vi "AlliGator Get Python Function Parameter Values Dialog.vi"(8 "Error In":errorcluster, 10 "Parameters In":string[][](array[string]), 11 "Input Message":string) -> (0 "Error Out":errorcluster, 1 "Cancelled?":bool, 2 "Parameters Out":string[][](array[string]))   [LabVIEW 2021, in "AlliGator Python Plugins.lvlib"]
doc: "Dialog to allow user to enter python function parameters."
uses:
  AlliGator Python Plugins.lvlib
  <vilib>/Utility/error.llb/Error Cluster From Error Code.vi
  <vilib>/ErrorRing/Error Ring.xnode
panel:
  out "Message":string
  in  "Parameters":i32(listbox)
  in  "Cancel":bool
  in  "OK":bool
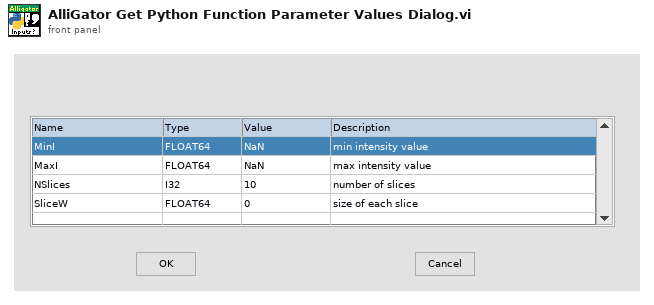
[diagram p1: front panel]
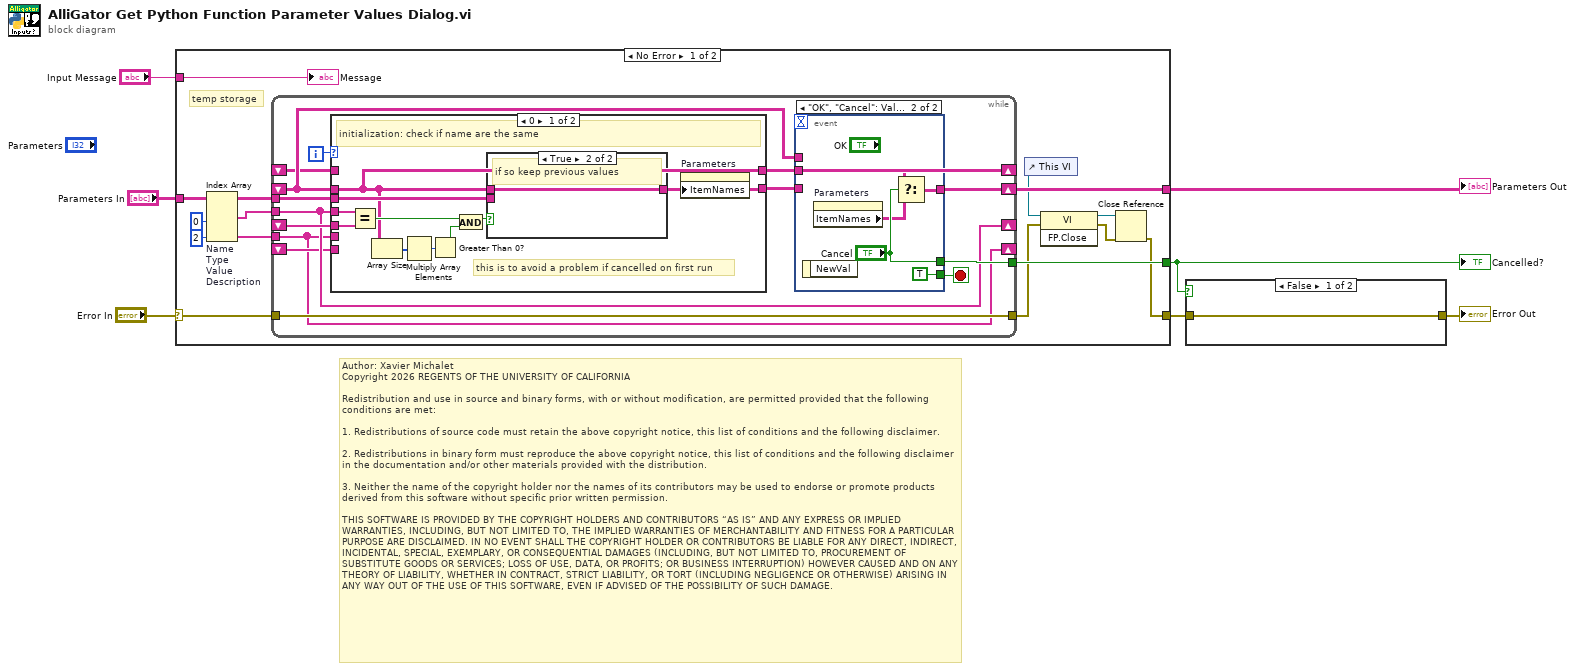
[diagram p0: block diagram]
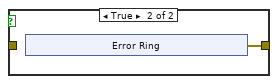
[diagram p2: hidden frame]
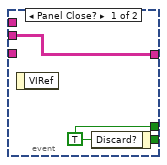
[diagram p5: hidden frame]
diagram:
  # "Author: Xavier Michalet\nCopyright 2026 REGENTS OF THE UNIVERSITY OF CALIFORNIA\n\nRedistribution and use in source and binary forms, with or without modification, are permitted provided that the following conditions are met:\n\n1. Redistributions of source code must retain the above copyright notice, this list of conditions and the following disclaimer.\n\n2. Redistributions in binary form must reproduce the above copyright notice, this list of conditions and the following disclaimer in the documentation and/or other materials provided with the distribution.\n\n3. Neither the name of the copyright holder nor the names of its contributors may be used to endorse or promote products derived from this software without specific prior written permission.\n\nTHIS SOFTWARE IS PROVIDED BY THE COPYRIGHT HOLDERS AND CONTRIBUTORS “AS IS” AND ANY EXPRESS OR IMPLIED WARRANTIES, INCLUDING, BUT NOT LIMITED TO, THE IMPLIED WARRANTIES OF MERCHANTABILITY AND FITNESS FOR A PARTICULAR PURPOSE ARE DISCLAIMED. IN NO EVENT SHALL THE COPYRIGHT HOLDER OR CONTRIBUTORS BE LIABLE FOR ANY DIRECT, INDIRECT, INCIDENTAL, SPECIAL, EXEMPLARY, OR CONSEQUENTIAL DAMAGES (INCLUDING, BUT NOT LIMITED TO, PROCUREMENT OF SUBSTITUTE GOODS OR SERVICES; LOSS OF USE, DATA, OR PROFITS; OR BUSINESS INTERRUPTION) HOWEVER CAUSED AND ON ANY THEORY OF LIABILITY, WHETHER IN CONTRACT, STRICT LIABILITY, OR TORT (INCLUDING NEGLIGENCE OR OTHERWISE) ARISING IN ANY WAY OUT OF THE USE OF THIS SOFTWARE, EVEN IF ADVISED OF THE POSSIBILITY OF SUCH DAMAGE."
  n1 = case shown="No Error" "Error In" {
    selector: "Error In" -> [w15 w57]
    tunnel: [w21 _] -> w3
    tunnel: [w20 _] -> w4
    tunnel: "Input Message" -> [w19 _]
    tunnel: [w16 w57] -> w2
    tunnel: "Parameters In" -> [w8 _]
    frame No Error {
      # "temp storage"
      n2 = Index Array "Name\nType\nValue\nDescription"(array=w8, index (col) #1=0 ("disabled index (col)"), index (col) #2=2 ("index (col)")) -> (element #1=w10:string[], element #2=w9:string[])  [unwired: 2 in]
      n3 = while {
        tunnel: [w34] -> w21
        shift-right: [w32] -> w20
        shift-left: _ -> [w27]
        tunnel: w15 -> [w30]
        tunnel: [w30] -> w14
        tunnel: w10 -> [w28]
        shift-right: [w28] -> _
        shift-left: _ -> [w29]
        tunnel: w9 -> [w25]
        shift-right: [w25] -> _
        shift-left: _ -> [w26]
        tunnel: w8 -> [w24]
        shift-right: [w22] -> _
        shift-left: _ -> [w23]
        i -> [w33]
        stop <- w35 stop-if-true
        n4 = case shown="0" w33 {
          tunnel: w27 -> [w40 w49]
          tunnel: [w42 w49] -> w31
          tunnel: w28 -> [w44 _]
          tunnel: w29 -> [w45 _]
          tunnel: w25 -> [_ _]
          tunnel: w26 -> [_ _]
          tunnel: w24 -> [w43 _]
          tunnel: [w40 w48] -> w22
          tunnel: w23 -> [_ w48]
          frame 0 {
            # "this is to avoid a problem if cancelled on first run"
            # "initialization: check if name are the same"
            n5 = Equal?(x=w44, y=w45) -> (x = y?=w41:bool)
            n6 = Array Size(array=w40) -> (size(s)=w39:i32[])
            n7 = Multiply Array Elements(1:w39) -> (0:w38:i32)
            n8 = Greater Than 0?(x=w38) -> (x > 0?=w36:bool)
            n9 = And(x=w41, y=w36) -> (x .and. y?=w37:bool)
            n10 = case shown="True" w37 {
              tunnel: w40 -> [_ w47]
              tunnel: [w46 w47] -> w42
              tunnel: w43 -> [w46 _]
              frame False {
                # "if not, use provided defaults"
              }
              frame True {
                # "if so keep previous values"
              }
            }
            n11 = property on="Parameters" class="MCListbox (strict)"("ItemNames"=w42) -> ()  [unwired: 2 in, 2 out]
          }
          frame 1, Default {
            # "subsequent events"
          }
        }
        n12 = event shown="[1] \"OK\", \"Cancel\": Value Change" {
          selector: _ -> [_ _]
          dyn-events: _ -> [_ _]
          timeout: _ -> [_ _]
          tunnel: [w51 TRUE ("Discard?")] -> w35
          tunnel: [w51 "Cancel"] -> w34
          tunnel: [w50 w54] -> w32
          tunnel: w31 -> [_ _]
          tunnel: w27 -> [_ _]
          tunnel: w22 -> [w50 w52]
          event Panel Close? {
            w51 = TRUE ("Discard?")
            n13 = event-data() -> ()  [unwired: 1 in, 1 out]
            n14 = event-data("Discard?"=w51) -> ()  [unwired: 1 in, 1 out]
          }
          event "OK", "Cancel": Value Change {
            n15 = event-data() -> ()  [unwired: 1 in, 1 out]
            n16 = property on="Parameters" class="MCListbox (strict)"() -> ("ItemNames"=w53:string[][])  [unwired: 2 in, 2 out]
            n17 = Select(t=w52, s="Cancel", f=w53) -> (s? t:f=w54:string[][])
          }
        }
      }
      n18 = control-ref of="This VI"() -> (w13:refnum<vi>)
      n19 = invoke class="VI" method="FP.Close"(reference=w13, error in=w14) -> (reference out=w18:refnum<vi>, error out=w17:errorcluster)  [unwired: 1 in, 1 out]
      n20 = Close Reference(reference=w18, error in (no error)=w17) -> (error out=w16:errorcluster)
      "Message" <- w19
    }
    frame Error {
    }
  }
  "Cancelled?" <- w3
  "Parameters Out" <- w4
  n21 = case shown="False" w3 {
    tunnel: w2 -> [w58 _]
    tunnel: [w58 w59] -> w1
    frame False {
    }
    frame True {
      n22 = xnode "Error Ring"() -> ("error out"=w59:errorcluster)
    }
  }
  "Error Out" <- w1
